vi "RS232ComPort WriteDeviceInfo.vi"(8 "error in (no error)":errorcluster, 9 "DeviceIndex":i32, 10 "DeviceInfo":T2, 11 "RS232ComPort in":refnum<class "RS232ComPort.lvclass">) -> (0 "error out":errorcluster, 3 "RS232ComPort out":refnum<class "RS232ComPort.lvclass">)   [LabVIEW 2018, in "RS232ComPort.lvclass"]
uses:
  RS232ComPort.lvclass
  RS232ComPort.lvclass/RS232ComPort.ctl
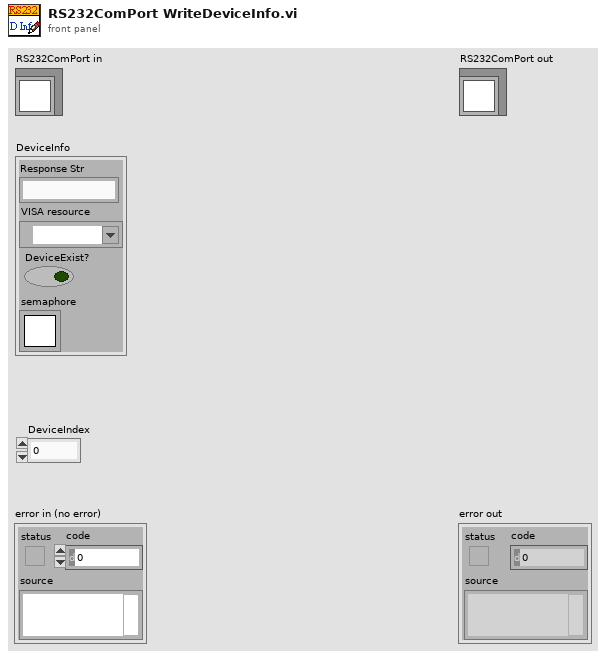
[diagram p1: front panel]
types:
  T1 = typedef "Semaphore RefNum" = refnum<k1>
  T2 = cluster{"Response Str":string, "VISA resource":refnum<visa-resource-name>, "DeviceExist?":bool, "semaphore":T1}
  T3 = cluster{"Response Str":string, "VISA resource":refnum<visa-resource-name>, "DeviceExist?":bool, "semaphore":T1}[]
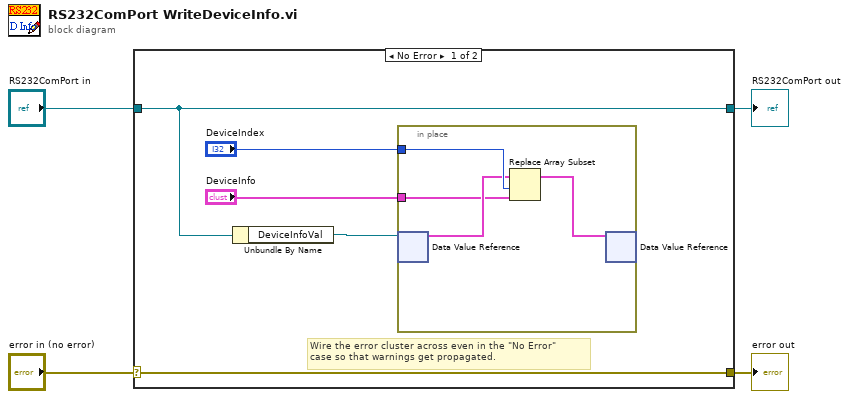
[diagram p0: block diagram]
diagram:
  n1 = case shown="No Error" "error in (no error)" {
    selector: "error in (no error)" -> [w9 w15]
    tunnel: [w9 w15] -> w3
    tunnel: [w8 w14] -> w1
    tunnel: "RS232ComPort in" -> [w8 w14]
    frame No Error {
      # "Wire the error cluster across even in the \"No Error\"\ncase so that warnings get propagated."
      n2 = Unbundle By Name(w8) -> ("DeviceInfoVal"=w7:refnum<data-value>)
      n3 = in-place {
        in-place-border: "DeviceIndex" -> [w13]
        in-place-border: "DeviceInfo" -> [w10]
        n4 = in-place-dvr #1(w7) -> (w11:T3)  [unwired: 1 out]
        n5 = Replace Array Subset(array=w11, new element=w10, index=w13) -> (w12:T3)
        n6 = in-place-dvr #1(w12) -> ()  [unwired: 2 out]
      }
    }
    frame Error {
    }
  }
  "error out" <- w3
  "RS232ComPort out" <- w1
